vi "Drive_Arcade.vi"(8 "error in":errorcluster, 9 "Y_Speed":dbl min=-1.0 max=1.0, 10 "X_Speed":dbl min=-1.0 max=1.0) -> (0 "error out":errorcluster)   [LabVIEW 2009, in "Drive.lvlib"]
doc: "This VI sets the speed vector for the robot. It requires two values for X and Y axes. \nThe range of both inputs is -1..+1, where -1 means max left value for X and max rear value for Y. +1 max right and max front correspondingly.\nFor example, to drive straight forward X_speed should be 0, and Y_speed should be >0.s"
uses:
  Drive.lvlib
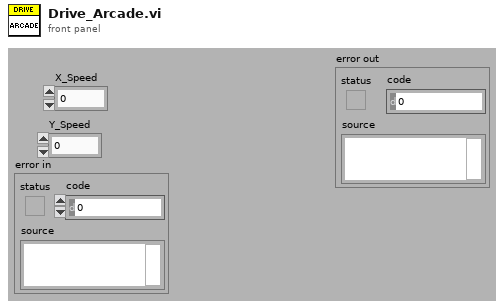
[diagram p1: front panel]
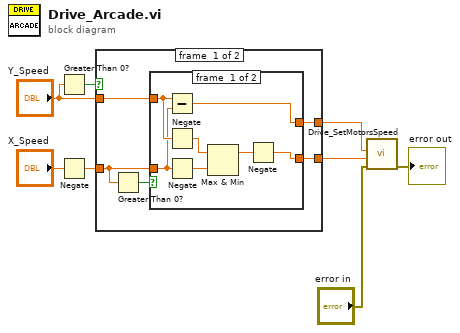
[diagram p0: block diagram]
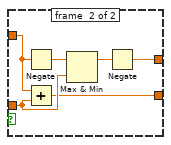
[diagram p2: hidden frame]
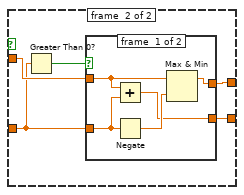
[diagram p3: hidden frame]
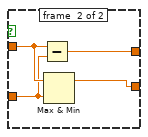
[diagram p4: hidden frame]
diagram:
  n1 = Greater Than 0?(x="Y_Speed") -> (x > 0?=w8:bool)
  n2 = Negate(x="X_Speed") -> (-x=w2:dbl)
  n3 = case shown="False" w8 {
    tunnel: "Y_Speed" -> [w12 w30]
    tunnel: w2 -> [w11 w29]
    tunnel: [w10 w28] -> w4
    tunnel: [w9 w27] -> w3
    frame #0 {
      n4 = Greater Than 0?(x=w11) -> (x > 0?=w13:bool)
      n5 = case shown="False" w13 {
        tunnel: w12 -> [w19 w25]
        tunnel: w11 -> [w17 w24]
        tunnel: [w14 w23] -> w9
        tunnel: [w20 w21] -> w10
        frame #0 {
          n6 = Subtract(x=w19, y=w17) -> (x-y=w20:dbl)
          n7 = Negate(x=w19) -> (-x=w18:dbl)
          n8 = Negate(x=w17) -> (-x=w16:dbl)
          n9 = Max & Min(x=w18, y=w16) -> (max(x,y)=w15:dbl)  [unwired: 1 out]
          n10 = Negate(x=w15) -> (-x=w14:dbl)
        }
        frame #1 {
          n11 = Negate(x=w25) -> (-x=w26:dbl)
          n12 = Add(x=w25, y=w24) -> (x+y=w23:dbl)
          n13 = Max & Min(x=w26, y=w24) -> (max(x,y)=w22:dbl)  [unwired: 1 out]
          n14 = Negate(x=w22) -> (-x=w21:dbl)
        }
      }
    }
    frame #1 {
      n15 = Greater Than 0?(x=w29) -> (x > 0?=w31:bool)
      n16 = case shown="False" w31 {
        tunnel: w30 -> [w34 w39]
        tunnel: w29 -> [w33 w38]
        tunnel: [w35 w40] -> w28
        tunnel: [w32 w37] -> w27
        frame #0 {
          n17 = Add(x=w34, y=w33) -> (x+y=w32:dbl)
          n18 = Negate(x=w33) -> (-x=w36:dbl)
          n19 = Max & Min(x=w34, y=w36) -> (max(x,y)=w35:dbl)  [unwired: 1 out]
        }
        frame #1 {
          n20 = Subtract(x=w39, y=w38) -> (x-y=w40:dbl)
          n21 = Max & Min(x=w39, y=w38) -> (max(x,y)=w37:dbl)  [unwired: 1 out]
        }
      }
    }
  }
  n22 = call "Drive_SetMotorsSpeed.vi"("error in"="error in", "Right_Speed"=w3, "Left_Speed"=w4) -> ("error out"=→"error out":errorcluster)  [unwired: 8 in]
